vi "DSF.Engine.Transceiver Thread.Transfer Group.Obtain.vi"(8 "error in (no error)":errorcluster, 10 "command parameters":T1, 11 "Transceiver Thread in":refnum<class "DSF.Engine.Transceiver Thread.lvclass">) -> (0 "error out":errorcluster, 2 "Transfer Group":refnum<class "DSF.Engine.Transfer Group.lvclass">, 3 "Transceiver Thread out":refnum<class "DSF.Engine.Transceiver Thread.lvclass">)   [LabVIEW 2017, in "Data Sharing Framework Engine.lvlib" / "DSF.Engine.Transceiver Thread.lvclass"]
uses:
  DSF.Engine.Transceiver Thread.lvclass
  Interface/DSF.Engine.Interface.Transceiver.Command Parameters.ctl
  Transfer/DSF.Engine.Transfer Group.lvclass
  DSF.Engine.Transceiver Thread.lvclass/DSF.Engine.Transceiver Thread.ctl
  Transfer/DSF.Engine.Transfer Group.lvclass/DSF.Engine.Transfer Group.ctl
  Timing/DSF.Engine.Timing.lvclass/DSF.Engine.Timing.ctl
  DSF.Engine.Transceiver Thread.Get Transfer Group.vi
  Transfer/DSF.Engine.Transfer Group.Get Timing.vi
  Timing/DSF.Engine.Timing.Iteration.Set.vi
  Transfer/DSF.Engine.Transfer Group.Set Timing.vi
  Timing/DSF.Engine.Timing.Set Iteration.vi
  Interface/DSF.Engine.Interface.Transceiver.lvclass
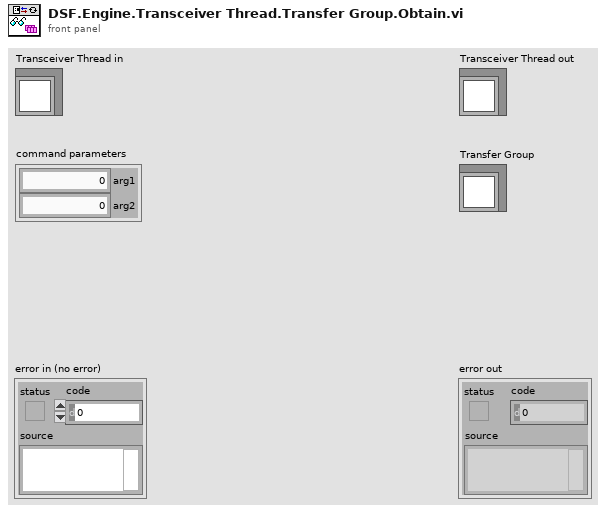
[diagram p1: front panel]
types:
  T1 = typedef "Data Sharing Framework Engine.lvlib/DSF.Engine.Interface.Transceiver.lvclass/DSF.Engine.Interface.Transceiver.Command Parameters.ctl" = cluster{"arg1":u64, "arg2":u64}
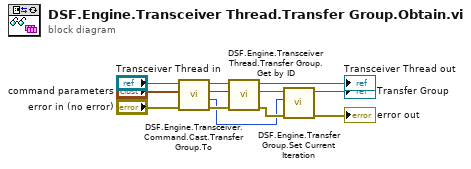
[diagram p0: block diagram]
diagram:
  n1 = call "DSF.Engine.Transceiver.Command.Cast.Transfer Group.To.vi"("error in (no error)"="error in (no error)", "command parameters"="command parameters", "Transceiver Thread in"="Transceiver Thread in") -> ("error out"=w10:errorcluster, "Transfer Group iteration"=w2:u64, "Transfer Group id"=w11:i32, "Transceiver Thread out"=w12:refnum<class "DSF.Engine.Transceiver Thread.lvclass">)  [unwired: 5 in]
  n2 = call "DSF.Engine.Transceiver Thread.Transfer Group.Get by ID.vi"("error in (no error)"=w10, "Transfer Group id"=w11, "Transceiver Thread in"=w12) -> ("error out"=w5:errorcluster, "Transfer Group"=w6:refnum<class "DSF.Engine.Transfer Group.lvclass">, "Transceiver Thread out"=→"Transceiver Thread out":refnum<class "DSF.Engine.Transceiver Thread.lvclass">)  [unwired: 6 in]
  n3 = call "DSF.Engine.Transfer Group.Set Current Iteration.vi"("error in (no error)"=w5, "iteration"=w2, "Transfer Group in"=w6) -> ("error out"=→"error out":errorcluster, "Transfer Group out"=→"Transfer Group":refnum<class "DSF.Engine.Transfer Group.lvclass">)  [unwired: 7 in]
